vi "XYZPosition.vi"(0 "VISA resource name":refnum<visa-resource-name>, 11 "error in":errorcluster) -> (4 "VISA resource name out":refnum<visa-resource-name>, 8 "[x,y,z]":dbl[](array[numeric]), 15 "error out":errorcluster)   [LabVIEW 2015]
doc: "This block outputs an array with the position of each axis. --Alex Kaufman"
uses:
  <userlib>/Newport ESP301/Newport ESP301.lvlib
panel:
  # "This outputs the position of each axis."
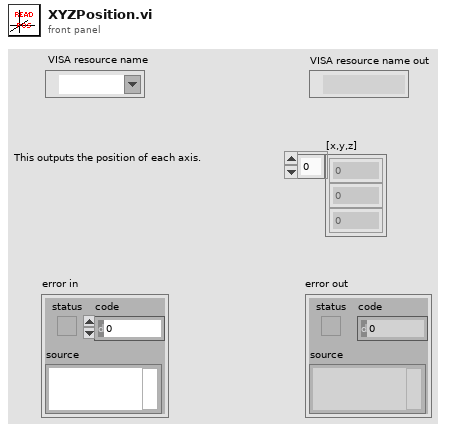
[diagram p1: front panel]
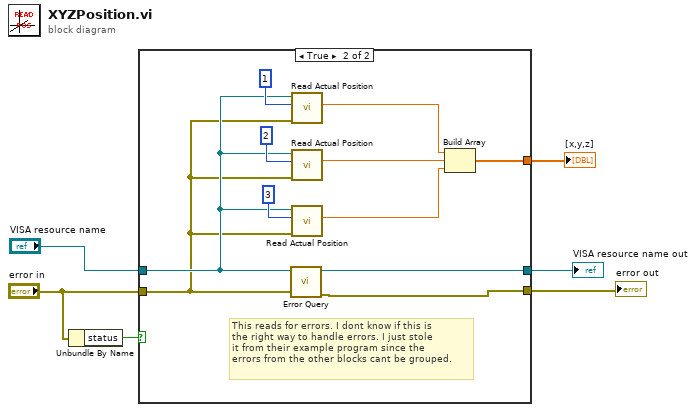
[diagram p0: block diagram]
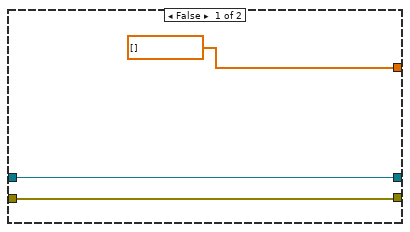
[diagram p2: hidden frame]
diagram:
  n1 = Unbundle By Name("error in") -> ("status"=w1:bool)
  n2 = case shown="True" w1 {
    tunnel: "VISA resource name" -> [w9 w17]
    tunnel: "error in" -> [w8 w16]
    tunnel: [w9 w12] -> w5
    tunnel: [w8 w11] -> w4
    tunnel: [dbl[] [] w10] -> w3
    frame False {
    }
    frame True {
      # "This reads for errors. I dont know if this is\nthe right way to handle errors. I just stole \nit from their example program since the \nerrors from the other blocks cant be grouped."
      n3 = call <userlib>:"Error Query.vi"("error in (no error)"=w16, "VISA resource name"=w17) -> ("error out"=w11:errorcluster, "VISA resource name out"=w12:refnum<visa-resource-name>)  [unwired: 2 in, 2 out]
      n4 = call <userlib>:"Read Actual Position.vi"("error in (no error)"=w16, "Axis (1)"=1, "VISA resource name"=w17) -> ("Position (units)"=w14:dbl)  [unwired: 2 in, 2 out]
      n5 = call <userlib>:"Read Actual Position.vi"("error in (no error)"=w16, "Axis (1)"=2, "VISA resource name"=w17) -> ("Position (units)"=w15:dbl)  [unwired: 2 in, 2 out]
      n6 = call <userlib>:"Read Actual Position.vi"("error in (no error)"=w16, "Axis (1)"=3, "VISA resource name"=w17) -> ("Position (units)"=w13:dbl)  [unwired: 2 in, 2 out]
      n7 = Build Array(w14, w15, w13) -> (w10:dbl[])
    }
  }
  "VISA resource name out" <- w5
  "error out" <- w4
  "[x,y,z]" <- w3
